vi "BuildTestFromProjectItem_LibraryWithUnsupportedTypes_BuildsEmptyTestSuite.vi"() -> ()   [LabVIEW 2017, in "LVUnitTestBuilder.Tests.lvlib"]
uses:
  LVUnitTestBuilder.Tests.lvlib
  LVUnitTestBuilder/LVUnitTestBuilder.lvclass
  Assertion/Assertion.lvlib
panel:
  out "error out":errorcluster
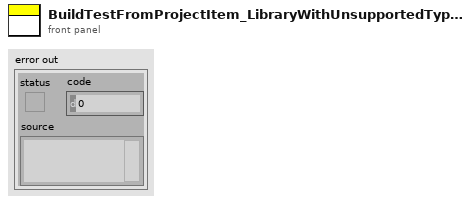
[diagram p1: front panel]
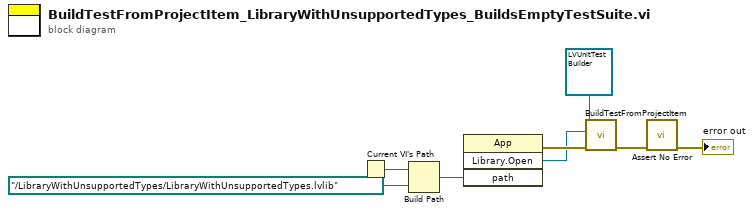
[diagram p0: block diagram]
diagram:
  n1 = Current VI's Path() -> (path=w4:path)
  n2 = Build Path(base path=w4, name or relative path=path "../LibraryWithUnsupportedTypes/LibraryWithUnsupportedTypes.lvlib") -> (appended path=w3:path)
  n3 = invoke class="App" method="Library.Open"("path"=w3) -> (error out=w7:errorcluster, "Open Library"=w6:refnum<vi>)  [unwired: 3 in, 2 out]
  n4 = call-dynamic "BuildTestFromProjectItem.vi"("error in (no error)"=w7, "ProjectItem Refnum"=w6, "LVUnitTestBuilder in"=refnum<class "LVUnitTestBuilder.lvclass"> refnum ("LVUnitTestBuilder")) -> ("error out"=w1:errorcluster)  [unwired: 6 in, 2 out]
  n5 = call "Assert No Error.vi"("error in (no error)"=w1) -> ("error out"=→"error out":errorcluster)  [unwired: 10 in]
